vi "Voltage_overflow_checker.vi"(2 "Voltages":dbl[][](array[numeric])) -> (0 "Over/Under string":string)   [LabVIEW 2010]
uses:
  Globals/Meas_global.vi
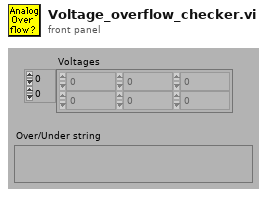
[diagram p1: front panel]
types:
  T1 = typedef "Board_Types.ctl" = enum16{"Simulate", "NB-MIO-16H", "PCI-MIO-16E", "6000E Series", "USB-92xx", "ADC488", "Lab-NB", "NB-DIO-24", "NI-DAQmx", "Local ADAM", "Server Channels"}
  T2 = typedef "Ch_and_Spans.ctl" = cluster{"high limit (10V)":sgl, "low limit (-10V)":sgl, "Ch No":i16, "Var name":string, "Use Latest Calib":bool}
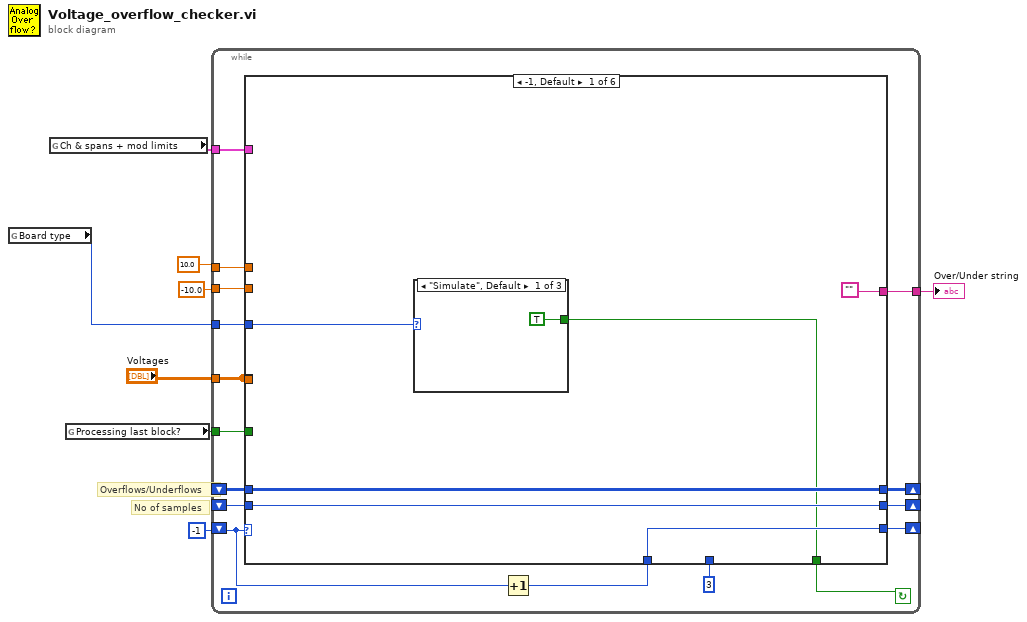
[diagram p0: block diagram]
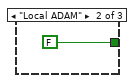
[diagram p2: hidden frame]
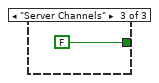
[diagram p3: hidden frame]
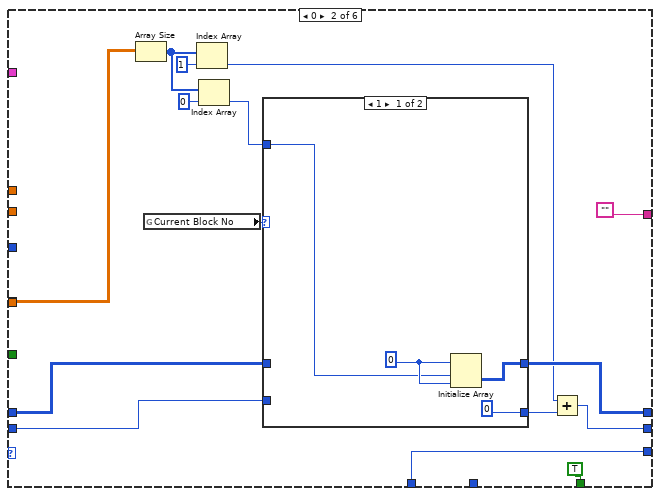
[diagram p4: hidden frame]
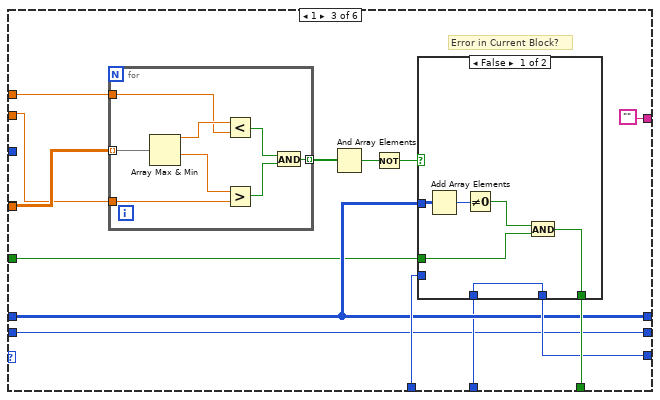
[diagram p6: hidden frame]
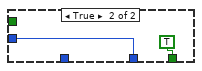
[diagram p7: hidden frame]
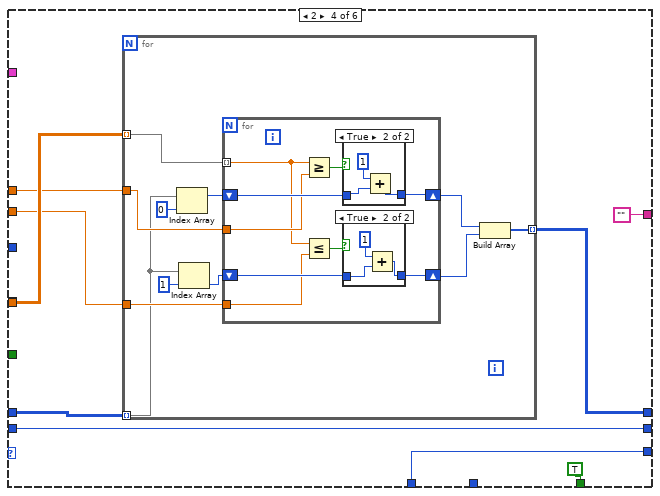
[diagram p8: hidden frame]
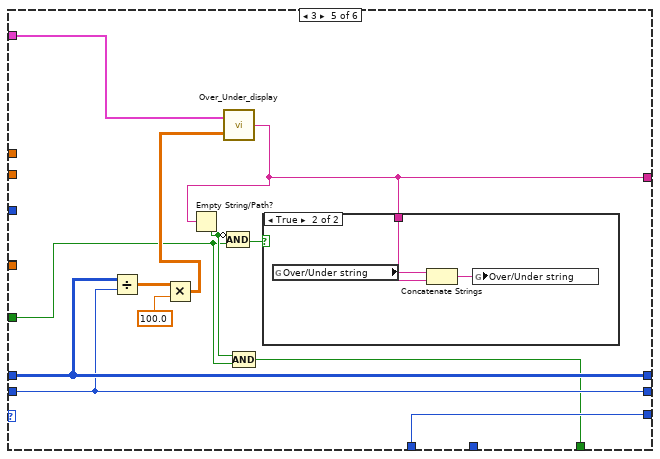
[diagram p11: hidden frame]
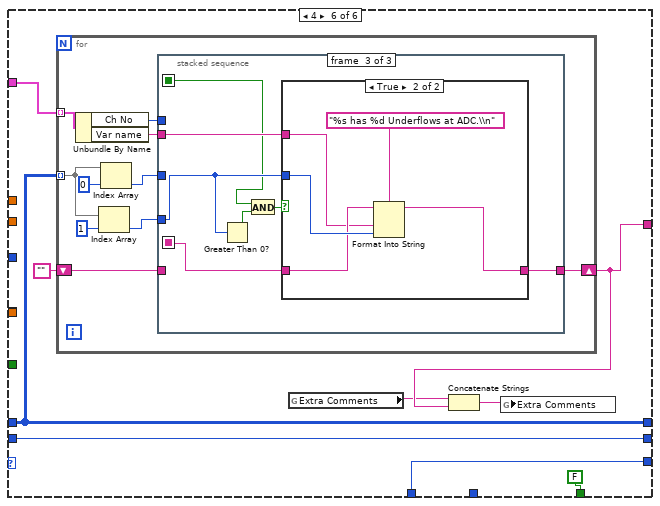
[diagram p13: hidden frame]
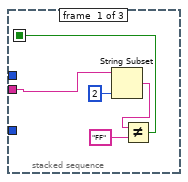
[diagram p14: hidden frame]
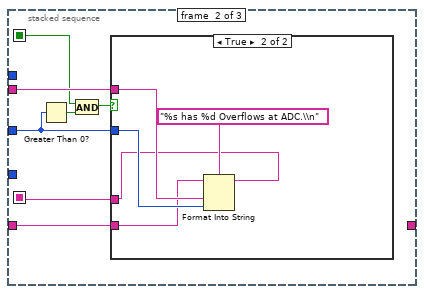
[diagram p15: hidden frame]
diagram:
  # "No of samples"
  # "Overflows/Underflows"
  n1 = global read "Meas_global.vi" "Board type"() -> (w4:T1)
  n2 = global read "Meas_global.vi" "Ch & spans + mod limits"() -> (w3:T2[])
  n3 = global read "Meas_global.vi" "Processing last block?"() -> (w6:bool)
  n4 = while {
    tunnel: w4 -> [w9]
    tunnel: [w10] -> w5
    tunnel: w6 -> [w12]
    shift-left: _ -> [w16]
    shift-right: [w13] -> _
    shift-left: _ -> [w15]
    shift-right: [w14] -> _
    tunnel: "Voltages" -> [w17]
    shift-left: -1 -> [w20]
    shift-right: [w18] -> _
    tunnel: -10.0 -> [w22]
    tunnel: 10.0 -> [w23]
    tunnel: w3 -> [w24]
    stop <- w21 continue-if-true
    n5 = Increment(x=w20) -> (x+1=w19:i32)
    n6 = case shown="-1, Default" w20 {
      tunnel: w24 -> [_ _ _ _ w132 w140]
      tunnel: w23 -> [_ _ w67 w91 _ _]
      tunnel: w22 -> [_ _ w66 w92 _ _]
      tunnel: w17 -> [_ w40 w68 _ _ _]
      tunnel: [w25 TRUE w63 TRUE w122 FALSE] -> w21
      tunnel: w19 -> [w27 w43 w61 w89 w133 w145]
      tunnel: [w27 w43 w62 w89 w133 w145] -> w18
      tunnel: w17 -> [_ _ _ w93 _ _]
      tunnel: w16 -> [w28 w46 w57 w85 w130 w144]
      tunnel: w15 -> [w29 w44 w60 w86 w131 w141]
      tunnel: [w29 w47 w60 w90 w131 w141] -> w14
      tunnel: [w28 w37 w57 w85 w130 w144] -> w13
      tunnel: w12 -> [_ _ w55 _ w123 _]
      tunnel: 3 -> [_ _ w59 _ _ _]
      tunnel: ["" "" "" "" w125 w138] -> w10
      tunnel: w9 -> [w26 _ _ _ _ _]
      frame -1, Default {
        n7 = case shown="\"Simulate\", Default" w26 {
          tunnel: [TRUE FALSE FALSE] -> w25
          frame "Simulate", Default {
          }
          frame "Local ADAM" {
          }
          frame "Server Channels" {
          }
        }
      }
      frame 0 {
        n8 = Array Size(array=w40) -> (size(s)=w35:i32[])
        n9 = global read "Meas_global.vi" "Current Block No"() -> (w48:i32)
        n10 = Index Array(array=w35, index=1 ("Index")) -> (element=w39:i32)
        n11 = Index Array(array=w35, index=0 ("Index")) -> (element=w34:i32)
        n12 = case shown="1" w48 {
          tunnel: [w52 w54] -> w47
          tunnel: w44 -> [_ w54]
          tunnel: w46 -> [_ w53]
          tunnel: [0 w53] -> w38
          tunnel: w34 -> [w49 _]
          frame 1 {
            w50 = 0
            n13 = Initialize Array(w50, w49, w50) -> (w52:i32[][])
          }
          frame 2, Default {
          }
        }
        n14 = Add(x=w39, y=w38) -> (x+y=w37:i32)
      }
      frame 1 {
        # "Error in Current Block?"
        n15 = for {
          tunnel: w68 -> [w84] mode=indexing
          tunnel: w67 -> [w82]
          tunnel: w66 -> [w80]
          tunnel: [w77] -> w65 mode=indexing
          n16 = Array Max & Min(array=w84) -> (max value=w83:dbl, min value=w81:dbl)  [unwired: 2 out]
          n17 = Less?(x=w83, y=w82) -> (x < y?=w78:bool)
          n18 = Greater?(x=w81, y=w80) -> (0:w79:bool)
          n19 = And(x=w78, y=w79) -> (x .and. y?=w77:bool)
        }
        n20 = And Array Elements(Boolean array=w65) -> (logical AND=w64:bool)
        n21 = Not(x=w64) -> (.not. x?=w56:bool)
        n22 = case shown="False" w56 {
          tunnel: [w70 TRUE] -> w63
          tunnel: [w69 w75] -> w62
          tunnel: w61 -> [_ w75]
          tunnel: w60 -> [w74 _]
          tunnel: w59 -> [w69 _]
          tunnel: w55 -> [w71 _]
          frame False {
            n23 = Add Array Elements(numeric array=w74) -> (sum=w73:i32)
            n24 = Not Equal To 0?(x=w73) -> (x != 0?=w72:bool)
            n25 = And(x=w72, y=w71) -> (x .and. y?=w70:bool)
          }
          frame True {
          }
        }
      }
      frame 2 {
        n26 = for {
          tunnel: w93 -> [w102] mode=indexing
          tunnel: w92 -> [w104]
          tunnel: w91 -> [w103]
          tunnel: [w100] -> w90 mode=indexing
          tunnel: w86 -> [w96] mode=indexing
          n27 = Index Array(array=w96, index=0 ("Index")) -> (element=w94:i32)
          n28 = Index Array(array=w96, index=1 ("Index")) -> (element=w95:i32)
          n29 = for {
            shift-right: [w108] -> w99
            shift-left: w95 -> [w109]
            shift-right: [w111] -> w101
            shift-left: w94 -> [w112]
            tunnel: w102 -> [w105] mode=indexing
            tunnel: w104 -> [w107]
            tunnel: w103 -> [w106]
            n30 = Greater Or Equal?(x=w105, y=w106) -> (x >= y?=w113:bool)
            n31 = Less Or Equal?(x=w105, y=w107) -> (x <= y?=w110:bool)
            n32 = case shown="True" w113 {
              tunnel: [w118 w120] -> w111
              tunnel: w112 -> [w118 w121]
              frame False {
              }
              frame True {
                n33 = Add(x=1, y=w121) -> (x+y=w120:i32)
              }
            }
            n34 = case shown="True" w110 {
              tunnel: w109 -> [w114 w116]
              tunnel: [w114 w115] -> w108
              frame False {
              }
              frame True {
                n35 = Add(x=1, y=w116) -> (x+y=w115:i32)
              }
            }
          }
          n36 = Build Array(w101, w99) -> (w100:i32[])
        }
      }
      frame 3 {
        n37 = Divide(x=w131, y=w130) -> (x/y=w129:dbl[][])
        n38 = Multiply(x=w129, y=100.0) -> (x*y=w127:dbl[][])
        n39 = call "Over_Under_display.vi"("Overflow array"=w127, "Ch & spans"=w132) -> ("Over/Under string"=w125:string)
        n40 = Empty String/Path?(string/path=w125) -> (empty?=w124:bool)
        n41 = Compound Arithmetic op=AND(invert w124, w123) -> (w126:bool)
        n42 = Compound Arithmetic op=AND(w124, w123) -> (w122:bool)
        n43 = case shown="True" w126 {
          tunnel: w125 -> [_ w134]
          frame False {
          }
          frame True {
            n44 = global read "Meas_global.vi" "Over/Under string"() -> (w136:string)
            n45 = Concatenate Strings(w136, w134) -> (w135:string)
            n46 = global write "Meas_global.vi" "Over/Under string"(w135) -> ()
          }
        }
      }
      frame 4 {
        n47 = for {
          tunnel: w140 -> [w155] mode=indexing
          tunnel: w141 -> [w154] mode=indexing
          shift-right: [w146] -> w138
          shift-left: "" -> [w147]
          n48 = Unbundle By Name(w155) -> ("Ch No"=w153:i16, "Var name"=w152:string)
          n49 = Index Array(array=w154, index=1) -> (element=w148:i32)
          n50 = Index Array(array=w154, index=0) -> (element=w149:i32)
          n51 = stacked-sequence {
            seq-local: [_ w165 _] -> [_ _ w180]
            seq-local: [w156 _ _] -> [_ w162 w174]
            tunnel: w148 -> [_ _ w178]
            tunnel: w149 -> [_ w164 _]
            tunnel: w152 -> [w157 w167 w177]
            tunnel: w153 -> [_ _ _]
            tunnel: w147 -> [_ w166 _]
            tunnel: [_ _ w179] -> w146
            frame #0 {
              n52 = String Subset(string=w157, length (rest)=2 ("length (rest)")) -> (substring=w159:string)  [unwired: 1 out]
              n53 = Not Equal?(x=w159, y="FF") -> (x != y?=w156:bool)
            }
            frame #1 {
              n54 = Greater Than 0?(x=w164) -> (x > 0?=w163:bool)
              n55 = And(x=w162, y=w163) -> (x .and. y?=w161:bool)
              n56 = case shown="True" w161 {
                tunnel: w164 -> [_ w171]
                tunnel: w167 -> [_ w172]
                tunnel: w166 -> [w168 w170]
                tunnel: [w168 w169] -> w165
                frame False {
                }
                frame True {
                  n57 = Format Into String(format string="%s has %d Overflows at ADC.\\n" ("Format String"), initial string=w170, w172, w171) -> (resulting string=w169:string)  [unwired: 1 in, 1 out]
                }
              }
            }
            frame #2 {
              n58 = Greater Than 0?(x=w178) -> (x > 0?=w176:bool)
              n59 = And(x=w174, y=w176) -> (x .and. y?=w175:bool)
              n60 = case shown="True" w175 {
                tunnel: w178 -> [_ w186]
                tunnel: w177 -> [_ w182]
                tunnel: w180 -> [w181 w185]
                tunnel: [w181 w184] -> w179
                frame False {
                }
                frame True {
                  n61 = Format Into String(format string="%s has %d Underflows at ADC.\\n" ("Format String"), initial string=w185, w182, w186) -> (resulting string=w184:string)  [unwired: 1 in, 1 out]
                }
              }
            }
          }
        }
        n62 = global read "Meas_global.vi" "Extra Comments"() -> (w137:string)
        n63 = Concatenate Strings(w137, w138) -> (w142:string)
        n64 = global write "Meas_global.vi" "Extra Comments"(w142) -> ()
      }
    }
  }
  "Over/Under string" <- w5
